vi "DAQmx Read (Analog 1D Wfm NChan NSamp).vi"(0 "task/channels in":refnum<k21>, 7 "number of samples per channel":i32=-1, 9 "timeout":dbl=10.0 format="%0.2f", 11 "error in":errorcluster) -> (4 "task out":refnum<k21>, 6 "data":waveform(dbl)[](array[waveform]), 15 "error out":errorcluster)   [LabVIEW 2011]
doc: "Reads one or more waveforms from a task that contains one or more analog input channels."
uses:
  nilvaiu.dll
panel:
  # "channel"
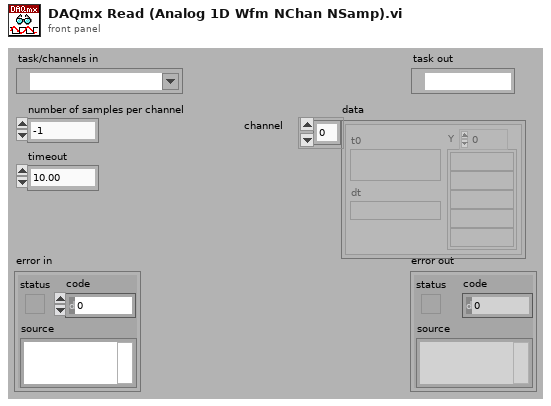
[diagram p1: front panel]
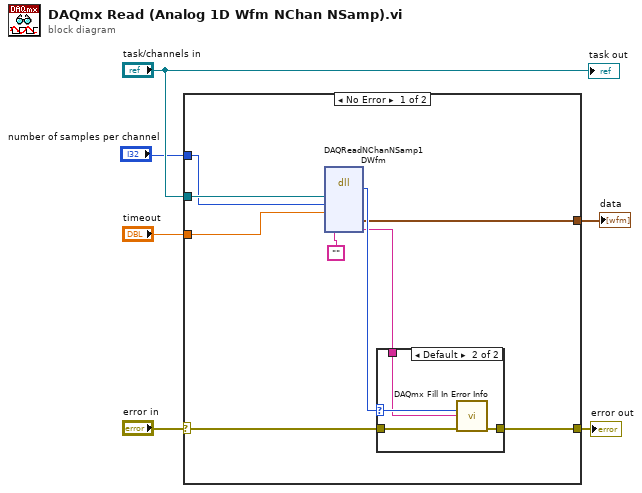
[diagram p0: block diagram]
diagram:
  n1 = case shown="No Error" "error in" {
    selector: "error in" -> [w9 w21]
    tunnel: [w14 w21] -> w5
    tunnel: "task/channels in" -> [w15 _]
    tunnel: [w10 _] -> w3
    tunnel: "timeout" -> [w8 _]
    tunnel: "number of samples per channel" -> [w7 _]
    frame No Error {
      n2 = dll-call lib="nilvaiu.*" fn="DAQReadNChanNSamp1DWfm"("taskID"=w15, "samplesPerCHannel"=w7, "timeout"=w8, "extendedErrorInfo"="") -> (w13:i32, "data"=w10:waveform(dbl)[], "extendedErrorInfo"=w11:string)  [unwired: 5 in, 4 out]
      n3 = case shown="Default" w13 {
        selector: w13 -> [_ w18]
        tunnel: w9 -> [w16 w20]
        tunnel: [w16 w19] -> w14
        tunnel: w11 -> [_ w17]
        frame 0 {
        }
        frame Default {
          n4 = call "DAQmx Fill In Error Info.vi"("status code"=w18, "extended error info"=w17, "error in"=w20) -> ("error out"=w19:errorcluster)  [unwired: 1 in, 11 out]
        }
      }
    }
    frame Error {
    }
  }
  "error out" <- w5
  "data" <- w3
  "task out" <- "task/channels in"
